vi "Bai1_4.vi"() -> ()   [LabVIEW 2018]
panel:
  out "Waveform Graph":dynamicdata(graph)
  in  "stop":bool
  in  "Enum":enum16{"Saw", "triangle", "sine"}(ring)
  in  "Noise amplitude":dbl=0.6
  in  "Phase":dbl
  in  "Amplitude":dbl=1.0
  in  "Frequency":dbl=10.1
  in  "Reset Signal":bool
  in  "Offset":dbl
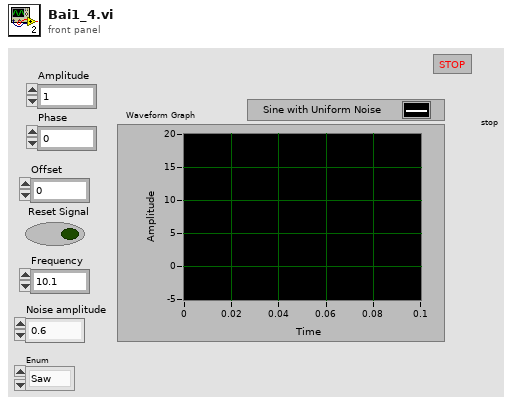
[diagram p1: front panel]
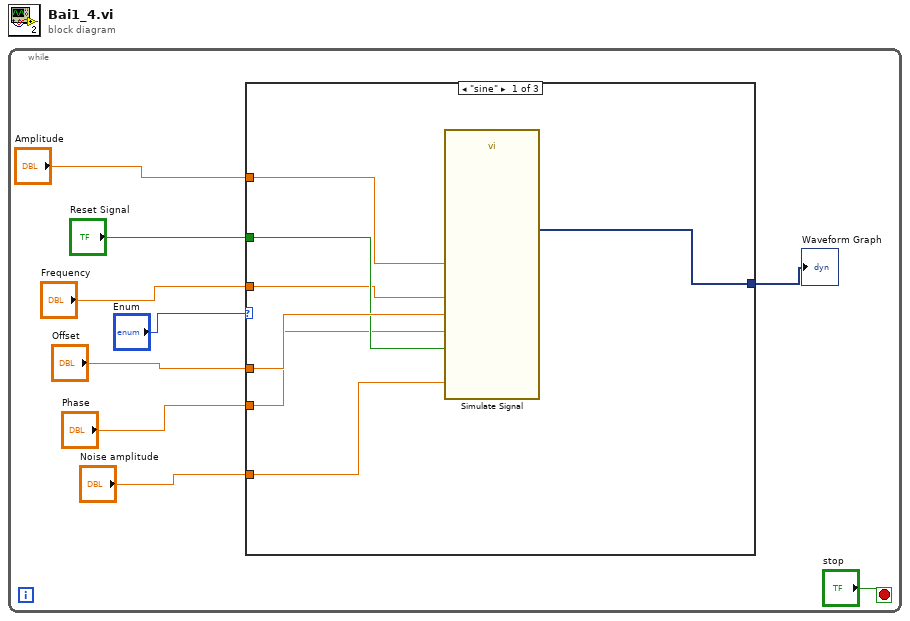
[diagram p0: block diagram]
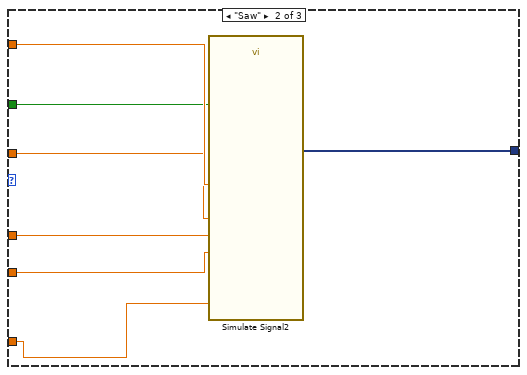
[diagram p2: hidden frame]
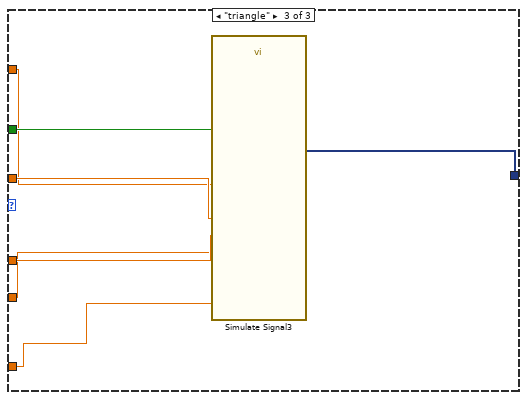
[diagram p3: hidden frame]
diagram:
  n1 = while {
    stop <- "stop" stop-if-true
    n2 = case shown="\"sine\"" "Enum" {
      tunnel: "Offset" -> [w16 w19 w28]
      tunnel: "Reset Signal" -> [w15 w22 w30]
      tunnel: "Frequency" -> [w14 w21 w29]
      tunnel: "Amplitude" -> [w13 w23 w25]
      tunnel: "Phase" -> [w12 w20 w26]
      tunnel: "Noise amplitude" -> [w11 w18 w27]
      tunnel: [w10 w17 w24] -> w1
      frame "sine" {
        n3 = call "Simulate Signal"("Offset"=w16, "Reset Signal"=w15, "Frequency"=w14, "Amplitude"=w13, "Phase"=w12, "Noise amplitude"=w11) -> ("Sine with Uniform Noise"=w10:dynamicdata)  [unwired: 8 in, 1 out]
      }
      frame "Saw" {
        n4 = call "Simulate Signal2"("Offset"=w19, "Reset Signal"=w22, "Frequency"=w21, "Amplitude"=w23, "Phase"=w20, "Noise amplitude"=w18) -> ("Sawtooth with Uniform Noise"=w17:dynamicdata)  [unwired: 8 in, 1 out]
      }
      frame "triangle" {
        n5 = call "Simulate Signal3"("Offset"=w28, "Reset Signal"=w30, "Frequency"=w29, "Amplitude"=w25, "Phase"=w26, "Noise amplitude"=w27) -> ("Triangle with Uniform Noise"=w24:dynamicdata)  [unwired: 8 in, 1 out]
      }
    }
    "Waveform Graph" <- w1
  }
